vi "Arduino COM Port Finder.vi"() -> (0 "Found com port? T/F":bool, 3 "Arduino Found COM port":string)   [LabVIEW 2021]
uses:
  <vilib>/Instr/_visa.llb/VISA Configure Serial Port (Instr).vi
panel:
  out "read buffer":string
  out "x = y?":bool
  out "error out":errorcluster
  out "concatenated string":string
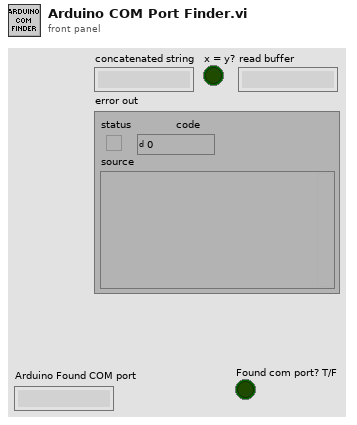
[diagram p1: front panel]
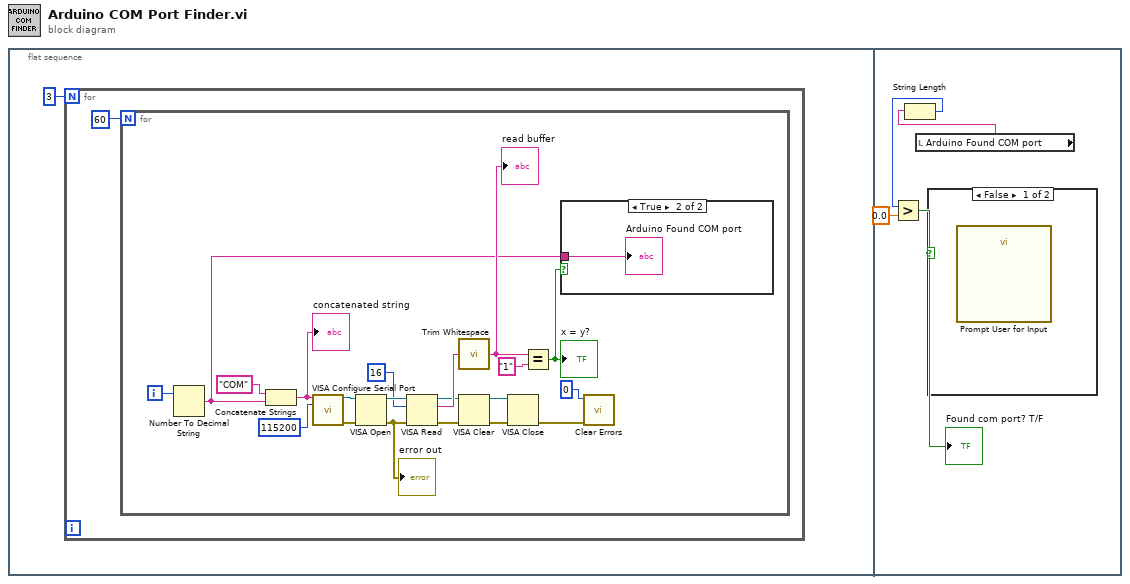
[diagram p0: block diagram]
diagram:
  n1 = flat-sequence {
    frame #0 {
      n2 = for {
        N: 3 -> [_]
        n3 = for {
          N: 60 -> [_]
          i -> [w5]
          n4 = Number To Decimal String(number=w5) -> (decimal integer string=w3:string)  [unwired: 1 in]
          n5 = Concatenate Strings("COM" ("string"), w3) -> (w21:string)
          "concatenated string" <- w21
          n6 = call-poly "VISA Configure Serial Port"("VISA resource name"=w21, "baud rate (9600)"=u32 115200) -> ("VISA resource name out"=w18:refnum<visa-resource-name>, "error out"=w17:errorcluster)  [unwired: 12 in]
          n7 = VISA Open(error in (no error)=w17, VISA resource name=w18) -> (VISA resource name=w8:refnum<visa-resource-name>, error out=w7:errorcluster)  [unwired: 3 in]
          "error out" <- w7
          n8 = VISA Read(VISA resource name=w8, byte count=u32 16, error in (no error)=w7) -> (VISA resource name out=w12:refnum<visa-resource-name>, read buffer=w16:string, error out=w9:errorcluster)  [unwired: 1 out]
          n9 = call <vilib>:"Trim Whitespace.vi"("string"=w16) -> ("trimmed string"=w15:string)  [unwired: 1 in]
          "read buffer" <- w15
          n10 = VISA Clear(VISA resource name=w12, error in (no error)=w9) -> (VISA resource name out=w11:refnum<visa-resource-name>, error out=w10:errorcluster)
          n11 = VISA Close(VISA resource name=w11, error in (no error)=w10) -> (error out=w13:errorcluster)
          n12 = Equal?(x=w15, y="1") -> (x = y?=w4:bool)
          "x = y?" <- w4
          n13 = case shown="True" w4 {
            tunnel: w3 -> [_ w23]
            frame False {
            }
            frame True {
              "Arduino Found COM port" <- w23
            }
          }
          n14 = call <vilib>:"Clear Errors.vi"("error in (no error)"=w13, "specific error code to clear (0: all)"=0) -> ()  [unwired: 4 in, 2 out]
        }
      }
    }
    frame #1 {
      n15 = local read "Arduino Found COM port"() -> (w27:string)
      n16 = String Length(string=w27) -> (length=w25:i32)
      n17 = Greater?(x=w25, y=0.0) -> (0:w24:bool)
      "Found com port? T/F" <- w24
      n18 = case shown="False" w24 {
        frame False {
          n19 = call "Prompt User for Input"() -> ()  [unwired: 18 in, 2 out]
        }
        frame True {
        }
      }
    }
  }
